vi "GOMDBTS2048 spectral Get Unit.vi"(8 "error in (no error)":errorcluster, 10 "calibrationEntryNumber":i32, 11 "handle":i32) -> (0 "error out":errorcluster, 2 "function return":i32, 3 "unit":string)   [LabVIEW 2015, in "GOMDBTS2048.lvlib"]
doc: "GOBTS2048DLL int __stdcall GOMDBTS2048_spectralGetUnit(int handle, int calibrationEntryNumber, char* unit);"
uses:
  GOMDBTS2048.lvlib
  runtime/GOMDBTS2048.dll
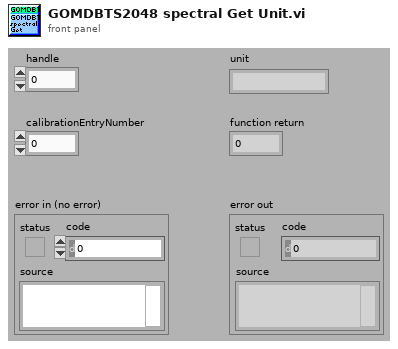
[diagram p1: front panel]
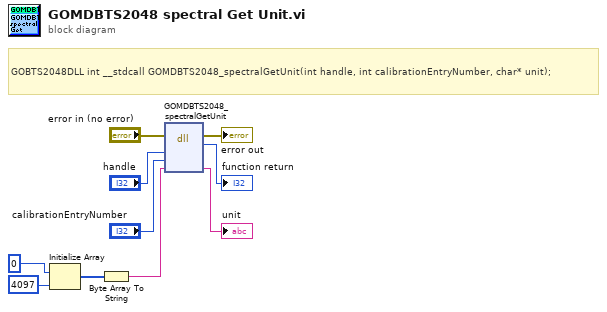
[diagram p0: block diagram]
diagram:
  # "GOBTS2048DLL int __stdcall GOMDBTS2048_spectralGetUnit(int handle, int calibrationEntryNumber, char* unit);"
  n1 = Initialize Array(u8 0 ("element"), 4097 ("dimension size")) -> (w7:u8[])
  n2 = Byte Array To String(unsigned byte array=w7) -> (string=w6:string)
  n3 = dll-call lib="C:/Users/rkoch/Documents/GO_Library/runtime/GOMDBTS2048.*" fn="GOMDBTS2048_spectralGetUnit"(error in="error in (no error)", "handle"="handle", "calibrationEntryNumber"="calibrationEntryNumber", "unit"=w6) -> (error out=→"error out":errorcluster, "return type"=→"function return":i32, "unit"=→"unit":string)  [unwired: 4 in, 1 out]
